vi "AutonIndex.vi"(4 "Intake Pressed":bool, 7 "Elevate Pressed":bool) -> (0 "Intake Arm":T1, 1 "Elevate":dbl, 2 "Reject":dbl, 3 "Intake":dbl)   [LabVIEW 2020]
uses:
  <vilib>/Rock Robotics/WPI/Solenoid/WPI_SolenoidValue.ctl
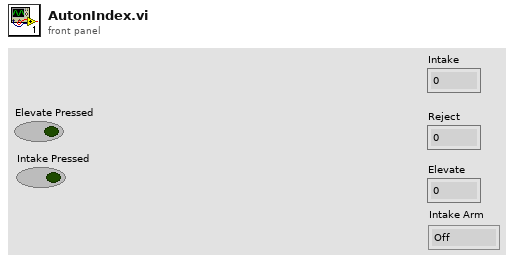
[diagram p1: front panel]
types:
  T1 = typedef "WPI_SolenoidValue.ctl" = enum16{"Off", "On", "Forward", "Reverse"}
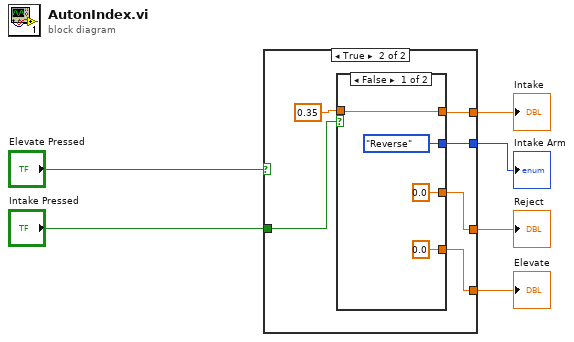
[diagram p0: block diagram]
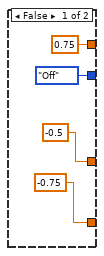
[diagram p2: hidden frame]
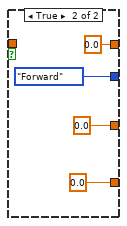
[diagram p3: hidden frame]
diagram:
  n1 = case shown="True" "Elevate Pressed" {
    tunnel: [0.75 ("Intake want") w14] -> w5
    tunnel: "Intake Pressed" -> [_ w16]
    tunnel: [WPI_SolenoidValue."Off" ("Intake Arm") w13] -> w3
    tunnel: [-0.5 ("Reject") w12] -> w2
    tunnel: [-0.75 ("Elevate") w11] -> w1
    frame False {
    }
    frame True {
      n2 = case shown="False" w16 {
        tunnel: [w20 0.0 ("Intake want")] -> w14
        tunnel: 0.35 ("Intake want") -> [w20 _]
        tunnel: [WPI_SolenoidValue."Reverse" ("Intake Arm") WPI_SolenoidValue."Forward" ("Intake Arm")] -> w13
        tunnel: [0.0 ("Reject") 0.0 ("Reject")] -> w12
        tunnel: [0.0 ("Elevate") 0.0 ("Elevate")] -> w11
        frame False {
        }
        frame True {
        }
      }
    }
  }
  "Intake" <- w5
  "Reject" <- w2
  "Elevate" <- w1
  "Intake Arm" <- w3
